vi "提取用户信息.vi"(8 "error in (no error)":errorcluster caption="错误输入（无错误）") -> (0 "error out":errorcluster caption="错误输出", 3 "用户信息":T1(array[cluster]))   [LabVIEW 2016, in "wxpusher.lvlib"]
uses:
  wxpusher.lvlib
  <vilib>/Utility/sysdir.llb/System Directory Type.ctl
  <vilib>/Utility/config.llb/Read Key (String).vi
  <vilib>/Utility/config.llb/NI_LVConfig.lvlib
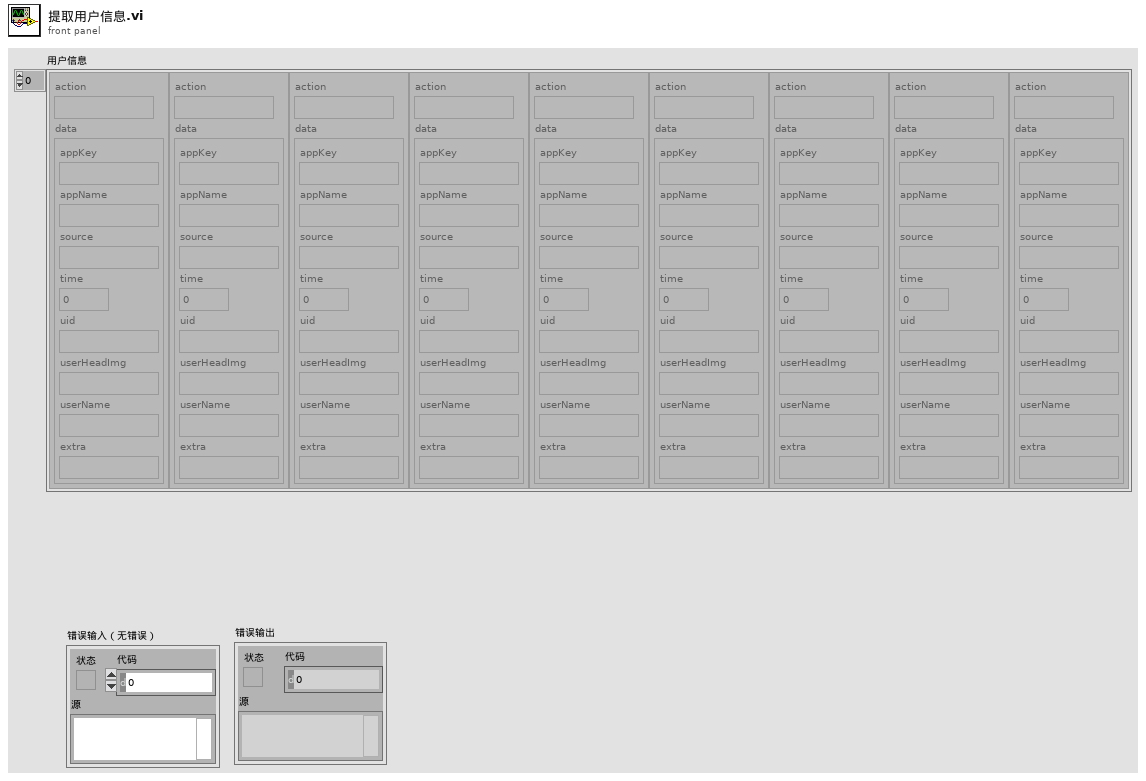
[diagram p1: front panel]
types:
  T1 = cluster{"action":string, "data":cluster{"appKey":string, "appName":string, "source":string, "time":u64, "uid":string, "userHeadImg":string, "userName":string, "extra":string}}[]
  T2 = typedef "System Directory Type.ctl" = i32
  T3 = typedef "NI_LVConfig.lvlib/Config Data RefNum.ctl" = refnum<k1>
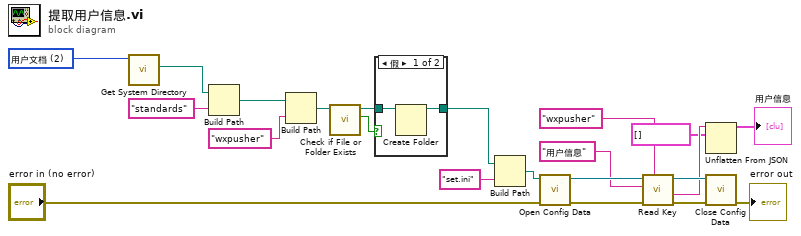
[diagram p0: block diagram]
diagram:
  w12 = T2 2 items=["用户目录"=0, "用户桌面"=1, "用户文档"=2, "用户应用程序数据"=3, "用户设置"=4, "用户临时目录"=5, "公共文档"=6, "公共应用程序数据"=7, "公共设置"=8, "公共缓存"=13, "系统核心库"=9, "系统安装库"=10, "应用程序文件"=11, "启动盘根目录"=12] ("system directory type")
  n1 = call <vilib>:"Get System Directory.vi"("system directory type"=w12) -> ("system directory"=w13:path)  [unwired: 10 in]
  n2 = Build Path(base path=w13, name or relative path="standards" ("名称或相对路径")) -> (appended path=w10:path)
  n3 = Build Path(base path=w10, name or relative path="wxpusher" ("名称或相对路径")) -> (appended path=w17:path)
  n4 = call <vilib>:"Check if File or Folder Exists.vi"("path"=w17) -> ("file or folder exists?"=w16:bool, "dup path"=w15:path)  [unwired: 8 in, 1 out]
  n5 = case shown="假" w16 {
    tunnel: w15 -> [w24 w25]
    tunnel: [w23 w25] -> w14
    frame False {
      n6 = Create Folder(path (use dialog)=w24) -> (created path=w23:path)  [unwired: 2 in, 2 out]
    }
    frame True {
    }
  }
  n7 = Build Path(base path=w14, name or relative path="set.ini" ("名称或相对路径")) -> (appended path=w21:path)
  n8 = call <vilib>:"Open Config Data.vi"("error in (no error)"="error in (no error)", "configuration file path"=w21) -> ("error out"=w8:errorcluster, "refnum"=w9:T3)  [unwired: 7 in, 1 out]
  n9 = call-poly <vilib>:"Read Key.vi"("section"="wxpusher", "error in (no error)"=w8, "key"="用户信息", "refnum"=w9) -> ("error out"=w6:errorcluster, "value"=w3:string, "refnum out"=w7:T3)  [unwired: 4 in, 1 out]
  n10 = Unflatten From JSON(JSON string=w3, type and defaults=T1 [] ("用户信息")) -> (value=→"用户信息":T1)  [unwired: 5 in, 1 out]
  n11 = call <vilib>:"Close Config Data.vi"("error in (no error)"=w6, "refnum"=w7) -> ("error out"=→"error out":errorcluster)  [unwired: 8 in, 1 out]
